vi "Gyro Veering V.5.0.vi"   [LabVIEW 2016]
uses:
  Robot Global Data V.5.0.vi
types:
  T1 = typedef "WPI_GyroDevRef.ctl" = cluster{"DevStatus":errorcluster, "Analog Channel":T2, "Offset":dbl, "Gain (VoltsPerDegree/Second)":dbl, "Gyro Type":enum16{"Analog", "XRS450"}, "Handle":i32, "SPI Bus":T3, "Device Found":bool, "Sample Rate":dbl, "Calibrate On Open":bool}
  T2 = typedef "FPGA_AIChannel.ctl" = enum8{"AI 0", "AI 1", "AI 2", "AI 3", "AI MXP 0", "AI MXP 1", "AI MXP 2", "AI MXP 3", "Invalid"}
  T3 = typedef "spi_bus.ctl" = enum16{"SPI On-Board, CS0", "SPI On-Board, CS1", "SPI On-Board, CS2", "SPI On-Board, CS3", "SPI MXP", "Invalid"}
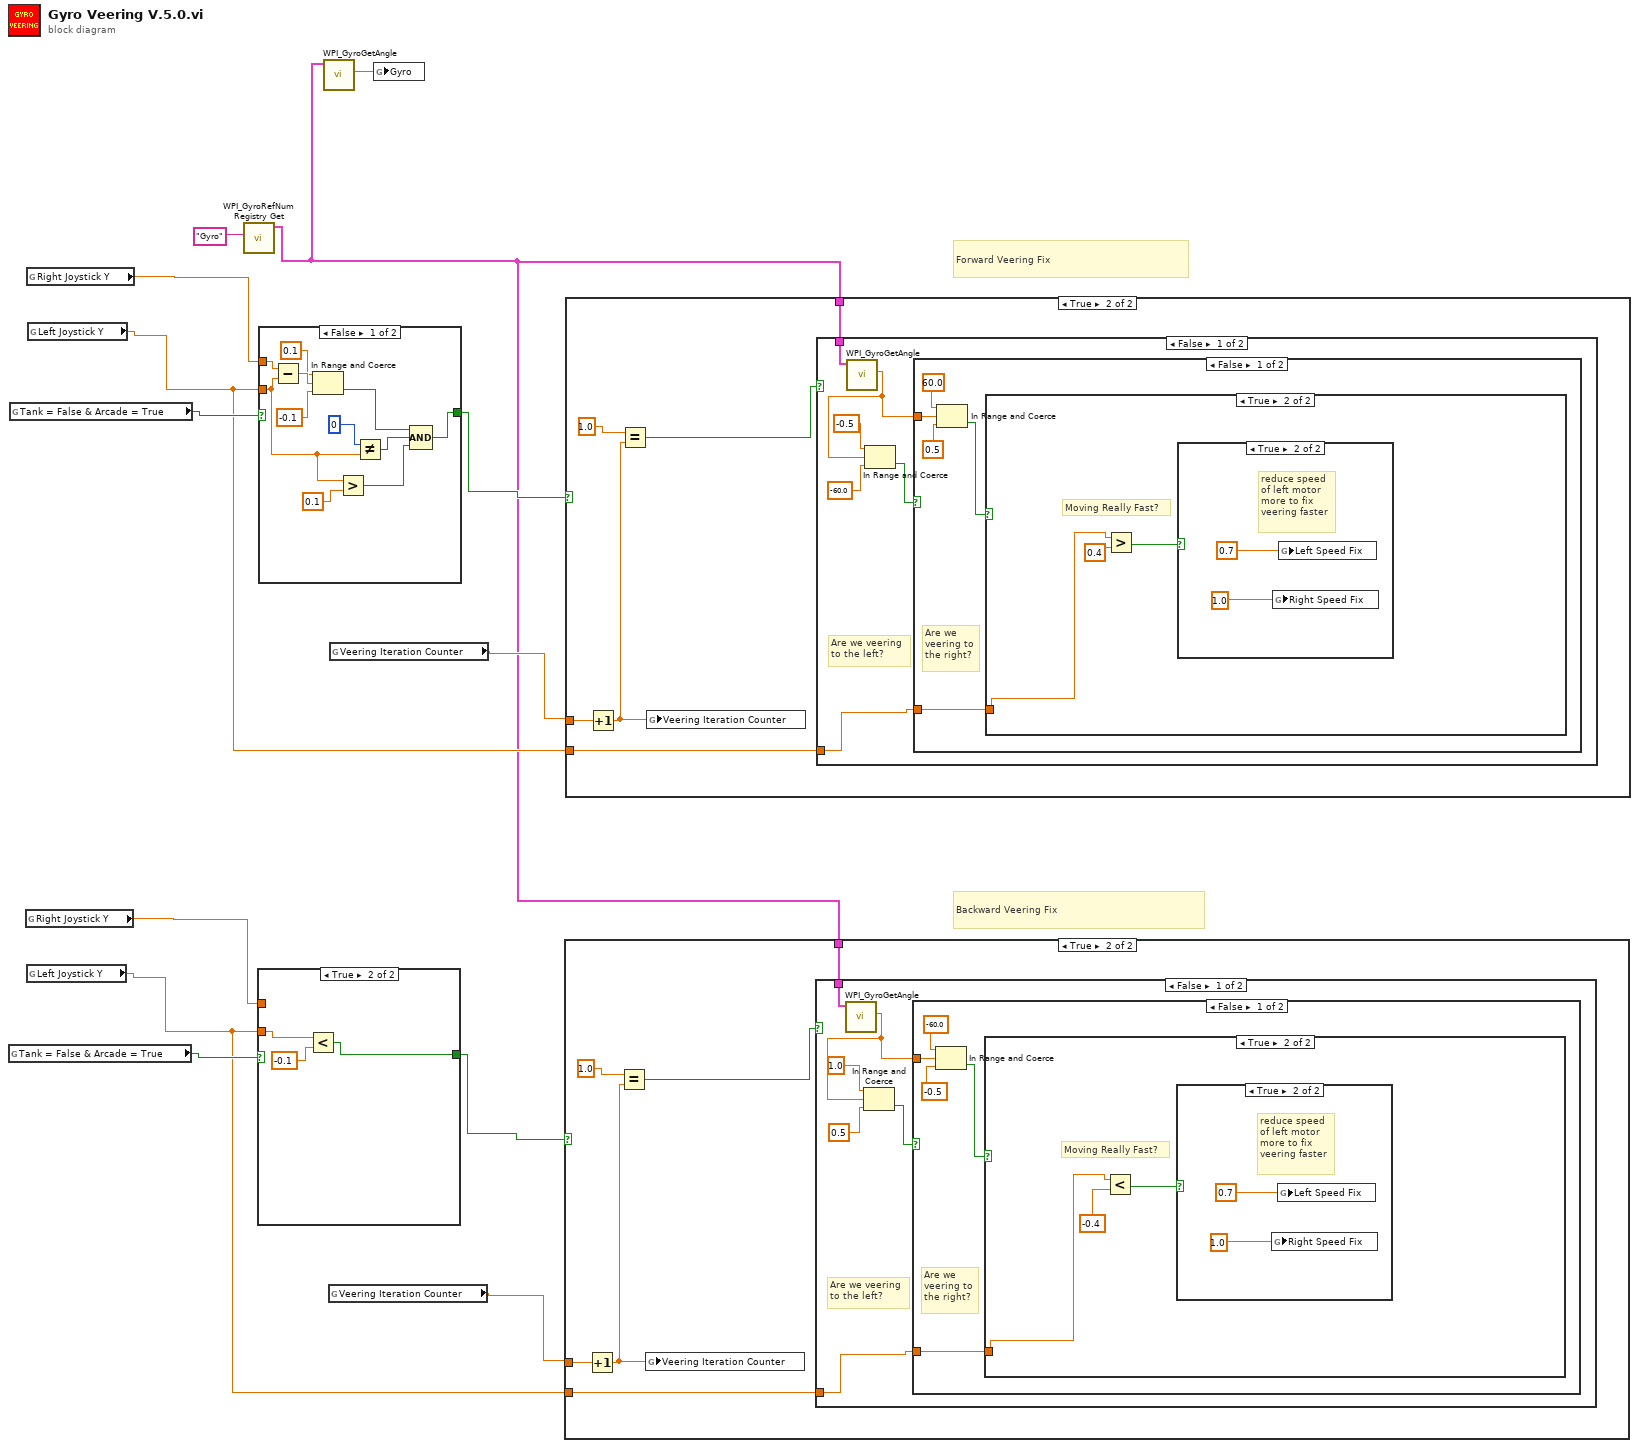
[diagram p0: block diagram]
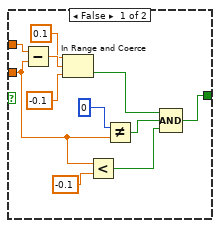
[diagram p2: hidden frame]
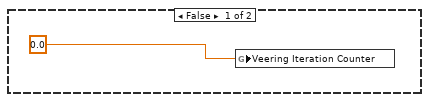
[diagram p3: hidden frame]
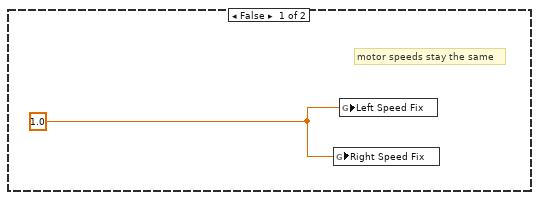
[diagram p4: hidden frame]
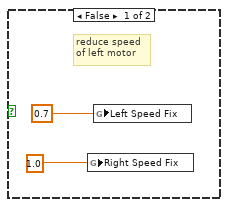
[diagram p5: hidden frame]
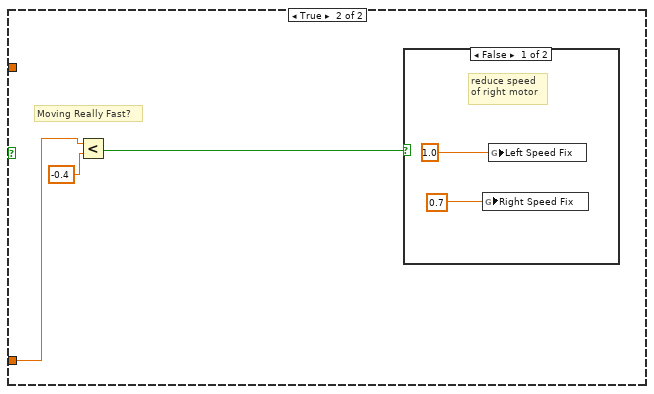
[diagram p6: hidden frame]
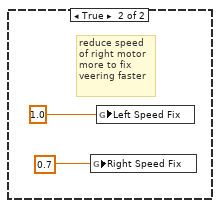
[diagram p7: hidden frame]
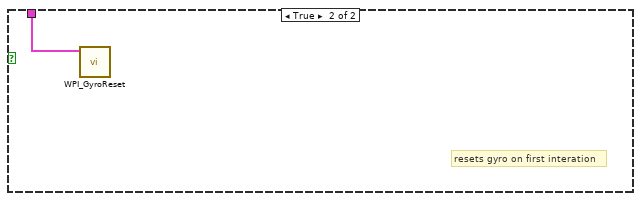
[diagram p8: hidden frame]
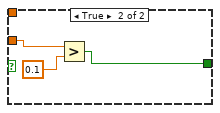
[diagram p9: hidden frame]
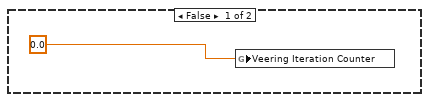
[diagram p10: hidden frame]
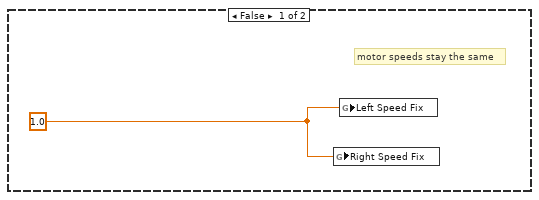
[diagram p11: hidden frame]
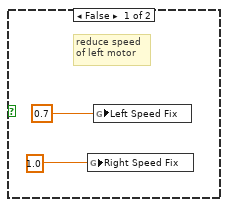
[diagram p12: hidden frame]
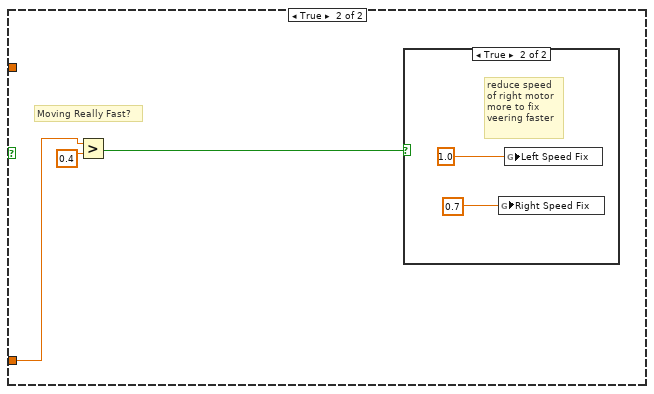
[diagram p13: hidden frame]
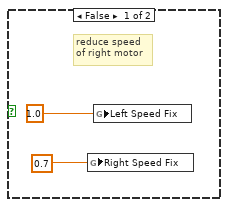
[diagram p14: hidden frame]
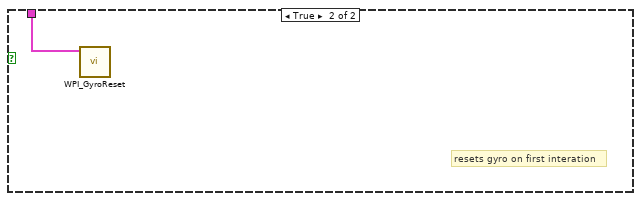
[diagram p15: hidden frame]
diagram:
  # "Backward Veering Fix"
  # "Forward Veering Fix"
  n1 = global read "Robot Global Data V.5.0.vi" "Tank = False & Arcade = True"() -> (w8:bool)
  n2 = global read "Robot Global Data V.5.0.vi" "Tank = False & Arcade = True"() -> (w13:bool)
  n3 = global read "Robot Global Data V.5.0.vi" "Right Joystick Y"() -> (w6:dbl)
  n4 = global read "Robot Global Data V.5.0.vi" "Right Joystick Y"() -> (w11:dbl)
  n5 = global read "Robot Global Data V.5.0.vi" "Left Joystick Y"() -> (w5:dbl)
  n6 = global read "Robot Global Data V.5.0.vi" "Left Joystick Y"() -> (w10:dbl)
  n7 = call <vilib>:"WPI_GyroRefNum Registry Get.vi"("refnum name"="Gyro") -> ("GyroDevRef"=w1:T1)  [unwired: 9 in, 1 out]
  n8 = case shown="True" w8 {
    tunnel: w5 -> [w16 w27]
    tunnel: [w17 w25] -> w7
    tunnel: w6 -> [w21 _]
    frame False {
      n9 = Subtract(x=w21, y=w16) -> (x-y=w24:dbl)
      n10 = In Range and Coerce(upper limit=0.1, x=w24, lower limit=-0.1) -> (In Range?=w19:bool)  [unwired: 1 out]
      n11 = Less?(x=w16, y=-0.1) -> (x < y?=w14:bool)
      n12 = Not Equal?(x=0, y=w16) -> (x != y?=w18:bool)
      n13 = Compound Arithmetic op=AND(w19, w18, w14) -> (w17:bool)
    }
    frame True {
      n14 = Less?(x=w27, y=-0.1) -> (x < y?=w25:bool)
    }
  }
  n15 = case shown="False" w13 {
    tunnel: w10 -> [w30 w41]
    tunnel: [w31 w39] -> w12
    tunnel: w11 -> [w35 _]
    frame False {
      n16 = Subtract(x=w35, y=w30) -> (x-y=w38:dbl)
      n17 = In Range and Coerce(upper limit=0.1, x=w38, lower limit=-0.1) -> (In Range?=w33:bool)  [unwired: 1 out]
      n18 = Greater?(x=w30, y=0.1) -> (0:w28:bool)
      n19 = Not Equal?(x=0, y=w30) -> (x != y?=w32:bool)
      n20 = Compound Arithmetic op=AND(w33, w32, w28) -> (w31:bool)
    }
    frame True {
      n21 = Greater?(x=w41, y=0.1) -> (0:w39:bool)
    }
  }
  n22 = call <vilib>:"WPI_GyroGetAngle.vi"("GyroDevRef"=w1) -> ("Angle"=w2:dbl)  [unwired: 6 in, 4 out]
  n23 = global read "Robot Global Data V.5.0.vi" "Veering Iteration Counter"() -> (w4:dbl)
  n24 = global read "Robot Global Data V.5.0.vi" "Veering Iteration Counter"() -> (w9:dbl)
  n25 = global write "Robot Global Data V.5.0.vi" "Gyro"(w2) -> ()
  n26 = case shown="True" w7 {
    tunnel: w1 -> [_ w48]
    tunnel: w4 -> [_ w46]
    tunnel: w5 -> [_ w43]
    frame False {
      n27 = global write "Robot Global Data V.5.0.vi" "Veering Iteration Counter"(0.0) -> ()
    }
    frame True {
      n28 = Increment(x=w46) -> (x+1=w44:dbl)
      n29 = Equal?(x=1.0, y=w44) -> (x = y?=w45:bool)
      n30 = global write "Robot Global Data V.5.0.vi" "Veering Iteration Counter"(w44) -> ()
      n31 = case shown="False" w45 {
        tunnel: w48 -> [w54 w75]
        tunnel: w43 -> [w49 _]
        frame False {
          # "Are we veering\nto the left?"
          n32 = call <vilib>:"WPI_GyroGetAngle.vi"("GyroDevRef"=w54) -> ("Angle"=w50:dbl)  [unwired: 6 in, 4 out]
          n33 = In Range and Coerce(upper limit=1.0, x=w50, lower limit=0.5) -> (In Range?=w51:bool)  [unwired: 1 out]
          n34 = case shown="False" w51 {
            tunnel: w50 -> [w58 _]
            tunnel: w49 -> [w55 w70]
            frame False {
              # "Are we \nveering to\nthe right?"
              n35 = In Range and Coerce(upper limit=-60.0, x=w58, lower limit=-0.5) -> (In Range?=w56:bool)  [unwired: 1 out]
              n36 = case shown="True" w56 {
                tunnel: w55 -> [_ w61]
                frame False {
                  w60 = 1.0
                  # "motor speeds stay the same"
                  n37 = global write "Robot Global Data V.5.0.vi" "Right Speed Fix"(w60) -> ()
                  n38 = global write "Robot Global Data V.5.0.vi" "Left Speed Fix"(w60) -> ()
                }
                frame True {
                  # "Moving Really Fast?"
                  n39 = Less?(x=w61, y=-0.4) -> (x < y?=w62:bool)
                  n40 = case shown="True" w62 {
                    frame False {
                      # "reduce speed \nof left motor"
                      n41 = global write "Robot Global Data V.5.0.vi" "Right Speed Fix"(1.0) -> ()
                      n42 = global write "Robot Global Data V.5.0.vi" "Left Speed Fix"(0.7) -> ()
                    }
                    frame True {
                      # "reduce speed \nof left motor\nmore to fix\nveering faster"
                      n43 = global write "Robot Global Data V.5.0.vi" "Right Speed Fix"(1.0) -> ()
                      n44 = global write "Robot Global Data V.5.0.vi" "Left Speed Fix"(0.7) -> ()
                    }
                  }
                }
              }
            }
            frame True {
              # "Moving Really Fast?"
              n45 = Less?(x=w70, y=-0.4) -> (x < y?=w68:bool)
              n46 = case shown="False" w68 {
                frame False {
                  # "reduce speed \nof right motor"
                  n47 = global write "Robot Global Data V.5.0.vi" "Right Speed Fix"(0.7) -> ()
                  n48 = global write "Robot Global Data V.5.0.vi" "Left Speed Fix"(1.0) -> ()
                }
                frame True {
                  # "reduce speed \nof right motor\nmore to fix\nveering faster"
                  n49 = global write "Robot Global Data V.5.0.vi" "Right Speed Fix"(0.7) -> ()
                  n50 = global write "Robot Global Data V.5.0.vi" "Left Speed Fix"(1.0) -> ()
                }
              }
            }
          }
        }
        frame True {
          # "resets gyro on first interation"
          n51 = call <vilib>:"WPI_GyroReset.vi"("GyroDevRef"=w75) -> ()  [unwired: 9 in, 2 out]
        }
      }
    }
  }
  n52 = case shown="True" w12 {
    tunnel: w1 -> [_ w82]
    tunnel: w9 -> [_ w80]
    tunnel: w10 -> [_ w77]
    frame False {
      n53 = global write "Robot Global Data V.5.0.vi" "Veering Iteration Counter"(0.0) -> ()
    }
    frame True {
      n54 = Increment(x=w80) -> (x+1=w78:dbl)
      n55 = Equal?(x=1.0, y=w78) -> (x = y?=w79:bool)
      n56 = global write "Robot Global Data V.5.0.vi" "Veering Iteration Counter"(w78) -> ()
      n57 = case shown="False" w79 {
        tunnel: w82 -> [w88 w109]
        tunnel: w77 -> [w83 _]
        frame False {
          # "Are we veering\nto the left?"
          n58 = call <vilib>:"WPI_GyroGetAngle.vi"("GyroDevRef"=w88) -> ("Angle"=w84:dbl)  [unwired: 6 in, 4 out]
          n59 = In Range and Coerce(upper limit=-0.5, x=w84, lower limit=-60.0) -> (In Range?=w85:bool)  [unwired: 1 out]
          n60 = case shown="False" w85 {
            tunnel: w84 -> [w92 _]
            tunnel: w83 -> [w89 w104]
            frame False {
              # "Are we \nveering to\nthe right?"
              n61 = In Range and Coerce(upper limit=60.0, x=w92, lower limit=0.5) -> (In Range?=w90:bool)  [unwired: 1 out]
              n62 = case shown="True" w90 {
                tunnel: w89 -> [_ w95]
                frame False {
                  w94 = 1.0
                  # "motor speeds stay the same"
                  n63 = global write "Robot Global Data V.5.0.vi" "Right Speed Fix"(w94) -> ()
                  n64 = global write "Robot Global Data V.5.0.vi" "Left Speed Fix"(w94) -> ()
                }
                frame True {
                  # "Moving Really Fast?"
                  n65 = Greater?(x=w95, y=0.4) -> (0:w96:bool)
                  n66 = case shown="True" w96 {
                    frame False {
                      # "reduce speed \nof left motor"
                      n67 = global write "Robot Global Data V.5.0.vi" "Right Speed Fix"(1.0) -> ()
                      n68 = global write "Robot Global Data V.5.0.vi" "Left Speed Fix"(0.7) -> ()
                    }
                    frame True {
                      # "reduce speed \nof left motor\nmore to fix\nveering faster"
                      n69 = global write "Robot Global Data V.5.0.vi" "Right Speed Fix"(1.0) -> ()
                      n70 = global write "Robot Global Data V.5.0.vi" "Left Speed Fix"(0.7) -> ()
                    }
                  }
                }
              }
            }
            frame True {
              # "Moving Really Fast?"
              n71 = Greater?(x=w104, y=0.4) -> (0:w102:bool)
              n72 = case shown="True" w102 {
                frame False {
                  # "reduce speed \nof right motor"
                  n73 = global write "Robot Global Data V.5.0.vi" "Right Speed Fix"(0.7) -> ()
                  n74 = global write "Robot Global Data V.5.0.vi" "Left Speed Fix"(1.0) -> ()
                }
                frame True {
                  # "reduce speed \nof right motor\nmore to fix \nveering faster"
                  n75 = global write "Robot Global Data V.5.0.vi" "Right Speed Fix"(0.7) -> ()
                  n76 = global write "Robot Global Data V.5.0.vi" "Left Speed Fix"(1.0) -> ()
                }
              }
            }
          }
        }
        frame True {
          # "resets gyro on first interation"
          n77 = call <vilib>:"WPI_GyroReset.vi"("GyroDevRef"=w109) -> ()  [unwired: 9 in, 2 out]
        }
      }
    }
  }
